vi "Servo MSMT SpecAn Configure Measure Step.vi"(8 "error in (no error)":errorcluster, 9 "Standard":string, 11 "Servo MSMT in":refnum<class "Servo MSMT.lvclass">) -> (0 "error out":errorcluster, 3 "Servo MSMT out":refnum<class "Servo MSMT.lvclass">)   [LabVIEW 2018, in "Servo MSMT.lvlib" / "Servo MSMT.lvclass"]
uses:
  Servo MSMT.lvclass
  C:/Sequence Automation/Plugins/Measurement Interface.lvlibp/Measurement Interface.lvclass
  Plugins/Measurement Interface.lvlibp/Private Methods/Measurement Name/Read Measurement Name.vi
  Plugins/TestStand API Tools (TSAT).lvlibp/Step Actions/TSAT Step Actions.lvlib
  Plugins/Measurement Interface.lvlibp/Measurement Interface.lvclass
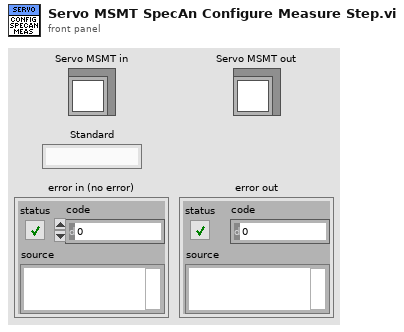
[diagram p1: front panel]
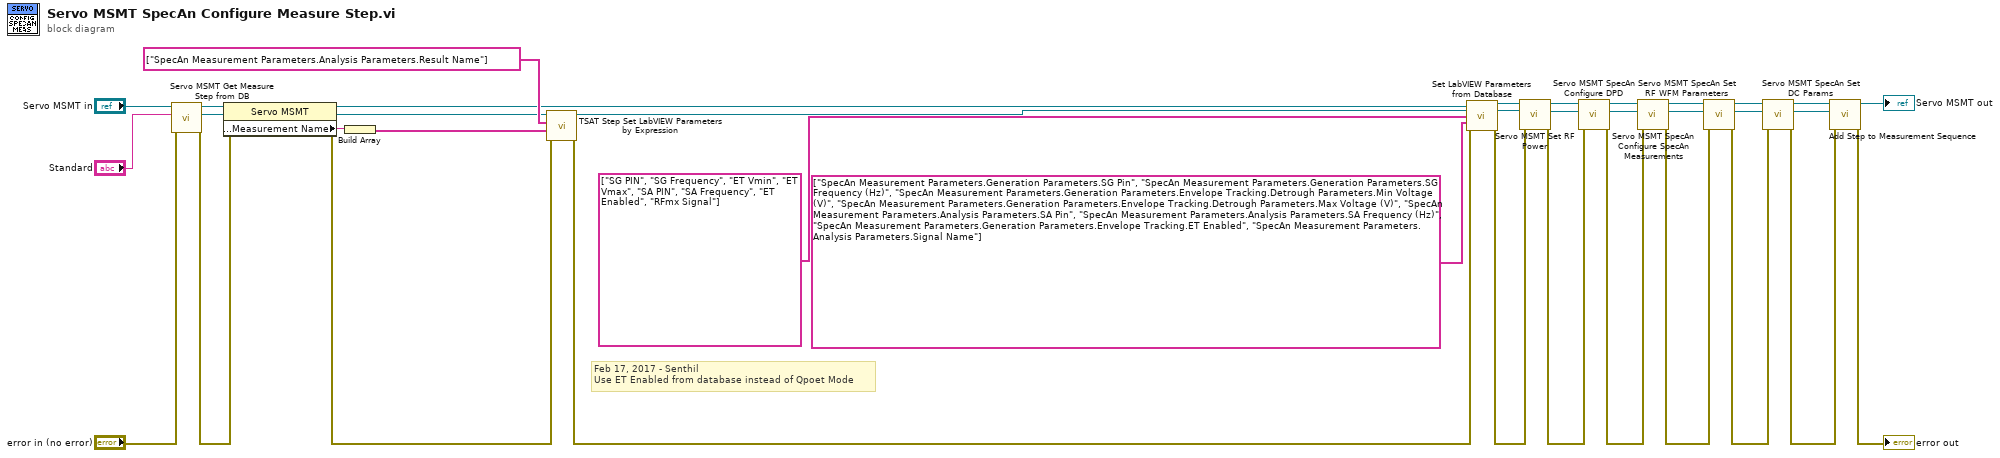
[diagram p0: block diagram]
diagram:
  # "Feb 17, 2017 - Senthil\nUse ET Enabled from database instead of Qpoet Mode"
  n1 = call "Servo MSMT Get Measure Step from DB.vi"("error in (no error)"="error in (no error)", "Standard"="Standard", "Servo MSMT in"="Servo MSMT in") -> ("error out"=w31:errorcluster, "Step Out"=w29:refnum<k7>, "Servo MSMT out"=w14:refnum<class "Servo MSMT.lvclass">)  [unwired: 6 in]
  n2 = property class="Servo MSMT"(reference=w14, error in=w31) -> (reference out=w13:refnum<class "Servo MSMT.lvclass">, error out=w15:errorcluster, "Public Methods:Measurement Name"=w12:string)
  n3 = Build Array(w12) -> (w34:string[])
  n4 = call "TSAT Step Set LabVIEW Parameters by Expression.vi"("Error In"=w15, "Value Expressions"=w34, "Parameters to Set"=string[] ["SpecAn Measurement Parameters.Analysis Parameters.Result Name"], "Step In"=w29) -> ("Error Out"=w32:errorcluster, "Step Out"=w30:refnum<k7>)  [unwired: 6 in]
  n5 = call "Set LabVIEW Parameters from Database.vi"("Measurement Interface in"=w13, "Step In"=w30, "Dictionary Keys"=string[] ["SG PIN", "SG Frequency", "ET Vmin", "ET Vmax", "SA PIN", "SA Frequency", "ET Enabled", "RFmx Signal"] ("Database Keys"), "LabVIEW Parameter Mapping"=string[] ["SpecAn Measurement Parameters.Generation Parameters.SG Pin", "SpecAn Measurement Parameters.Generation Parameters.SG Frequency (Hz)", "SpecAn Measurement Parameters.Generation Parameters.Envelope Tracking.Detrough Parameters.Min Voltage (V)", "SpecAn Measurement Parameters.Generation Parameters.Envelope Tracking.Detrough Parameters.Max Voltage (V)", "SpecAn Measurement Parameters.Analysis Parameters.SA Pin", "SpecAn Measurement Parameters.Analysis Parameters.SA Frequency (Hz)", "SpecAn Measurement Parameters.Generation Parameters.Envelope Tracking.ET Enabled", "SpecAn Measurement Parameters.Analysis Parameters.Signal Name"] ("Database Keys"), "error in (no error)"=w32) -> ("Measurement Interface out"=w10:refnum<class "Servo MSMT.lvclass">, "Step Out"=w9:refnum<k7>, "error out"=w20:errorcluster)  [unwired: 8 in]
  n6 = call-dynamic "Servo MSMT Set RF Power.vi"("error in (no error)"=w20, "Step In"=w9, "Servo MSMT in"=w10) -> ("error out"=w11:errorcluster, "Step Out"=w2:refnum<k7>, "Servo MSMT out"=w4:refnum<class "Servo MSMT.lvclass">)  [unwired: 6 in]
  n7 = call "Servo MSMT SpecAn Configure DPD.vi"("error in (no error)"=w11, "Step In"=w2, "Servo MSMT in"=w4) -> ("error out"=w5:errorcluster, "Step Out"=w1:refnum<k7>, "Servo MSMT out"=w3:refnum<class "Servo MSMT.lvclass">)  [unwired: 6 in]
  n8 = call "Servo MSMT SpecAn Configure SpecAn Measurements.vi"("error in (no error)"=w5, "Step In"=w1, "Servo MSMT in"=w3) -> ("error out"=w8:errorcluster, "Step Out"=w6:refnum<k7>, "Servo MSMT out"=w7:refnum<class "Servo MSMT.lvclass">)  [unwired: 6 in]
  n9 = call "Servo MSMT SpecAn Set RF WFM Parameters.vi"("error in (no error)"=w8, "Step In"=w6, "Servo MSMT in"=w7) -> ("error out"=w21:errorcluster, "Step Out"=w24:refnum<k7>, "Servo MSMT out"=w23:refnum<class "Servo MSMT.lvclass">)  [unwired: 6 in]
  n10 = call "Servo MSMT SpecAn Set DC Params.vi"("error in (no error)"=w21, "Step In"=w24, "Servo MSMT in"=w23) -> ("error out"=w22:errorcluster, "Step Out"=w28:refnum<k7>, "Servo MSMT out"=w26:refnum<class "Servo MSMT.lvclass">)  [unwired: 6 in]
  n11 = call "Add Step to Measurement Sequence.vi"("error in (no error)"=w22, "Step to Add"=w28, "Measurement Interface in"=w26) -> ("error out"=→"error out":errorcluster, "Measurement Interface out"=→"Servo MSMT out":refnum<class "Servo MSMT.lvclass">)  [unwired: 7 in]
